vi "Main.vi"() -> ()   [LabVIEW 2024, in "Application.lvclass"]
uses:
  Application.lvclass
  <vilib>/event_ctls.llb/usereventprio.ctl
panel:
  in  "Button 20":bool
  in  "Button 19":bool
  in  "Button 18":bool
  in  "Button 17":bool
  in  "Button 16":bool
  in  "Button 15":bool
  in  "Button 14":bool
  in  "Button 13":bool
  in  "Button 12":bool
  in  "Button 11":bool
  in  "Button 10":bool
  in  "Button 9":bool
  in  "Button 8":bool
  in  "Button 7":bool
  in  "Button 6":bool
  in  "Button 5":bool
  in  "Button 4":bool
  in  "Button 3":bool
  in  "Button 2":bool
  in  "Button":bool
  out "User":string
  in  "Failure":bool
  in  "Next":bool
  in  "Previous":bool
  in  "Last":bool
  in  "First":bool
  out "date/time string":string
  in  "Tab Control":enum32{"Thumbnails", "Full Image", "Failures"}(tab)
  out "2D Picture 35":picture
  out "2D Picture 34":picture
  out "2D Picture 33":picture
  out "2D Picture 32":picture
  out "2D Picture 31":picture
  out "2D Picture 30":picture
  out "2D Picture 29":picture
  out "2D Picture 28":picture
  out "2D Picture 27":picture
  out "2D Picture 26":picture
  out "2D Picture 25":picture
  out "2D Picture 24":picture
  out "2D Picture 23":picture
  out "2D Picture 22":picture
  out "2D Picture 21":picture
  out "2D Picture 20":picture
  out "2D Picture 19":picture
  out "2D Picture 18":picture
  out "2D Picture 17":picture
  out "2D Picture 16":picture
  out "2D Picture 15":picture
  out "2D Picture 14":picture
  out "2D Picture 13":picture
  out "2D Picture 12":picture
  out "2D Picture 11":picture
  out "2D Picture 10":picture
  out "2D Picture 9":picture
  out "2D Picture 8":picture
  out "2D Picture":picture
  out "2D Picture 2":picture
  out "2D Picture 3":picture
  out "2D Picture 4":picture
  out "2D Picture 5":picture
  out "2D Picture 6":picture
  out "2D Picture 7":picture
  out "FullSize":picture
  out "error out":errorcluster
  # "IMAGE ANALYSIS PROTOTYPE"
  # "Hit any key to stop program"
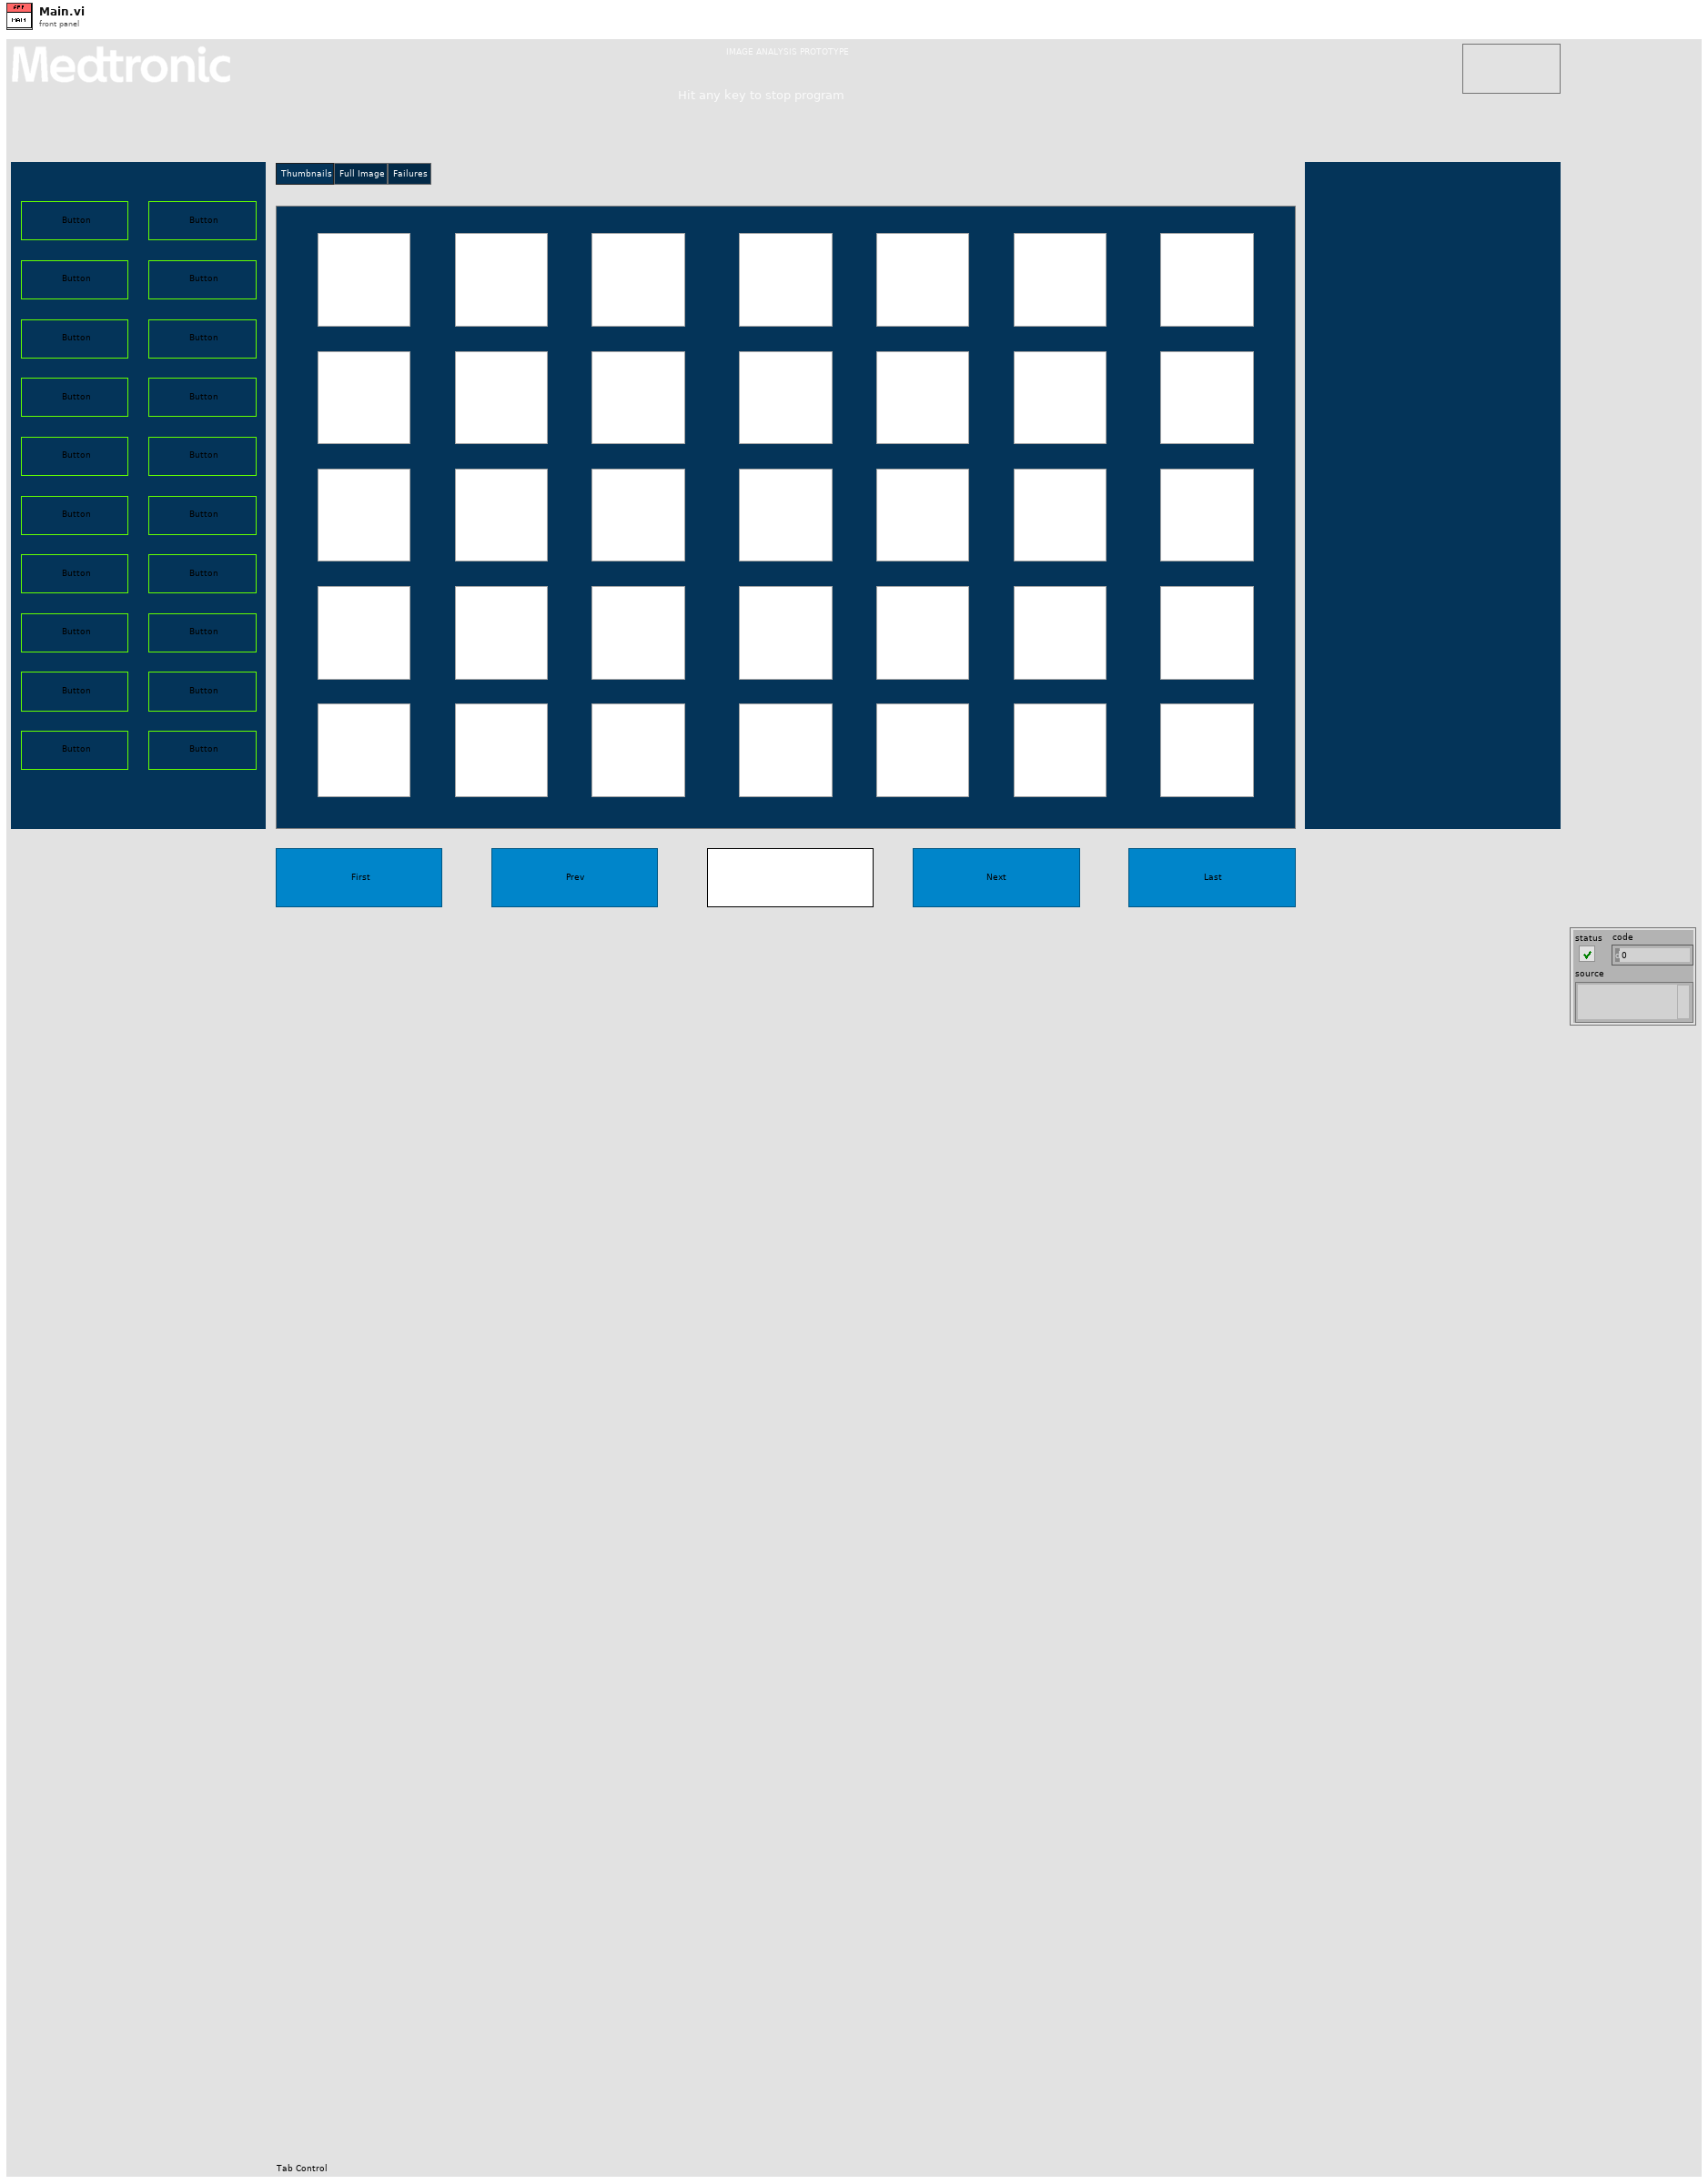
[diagram p1: front panel]
types:
  T1 = typedef "usereventprio.ctl" = enum32{"high priority", "normal priority"}
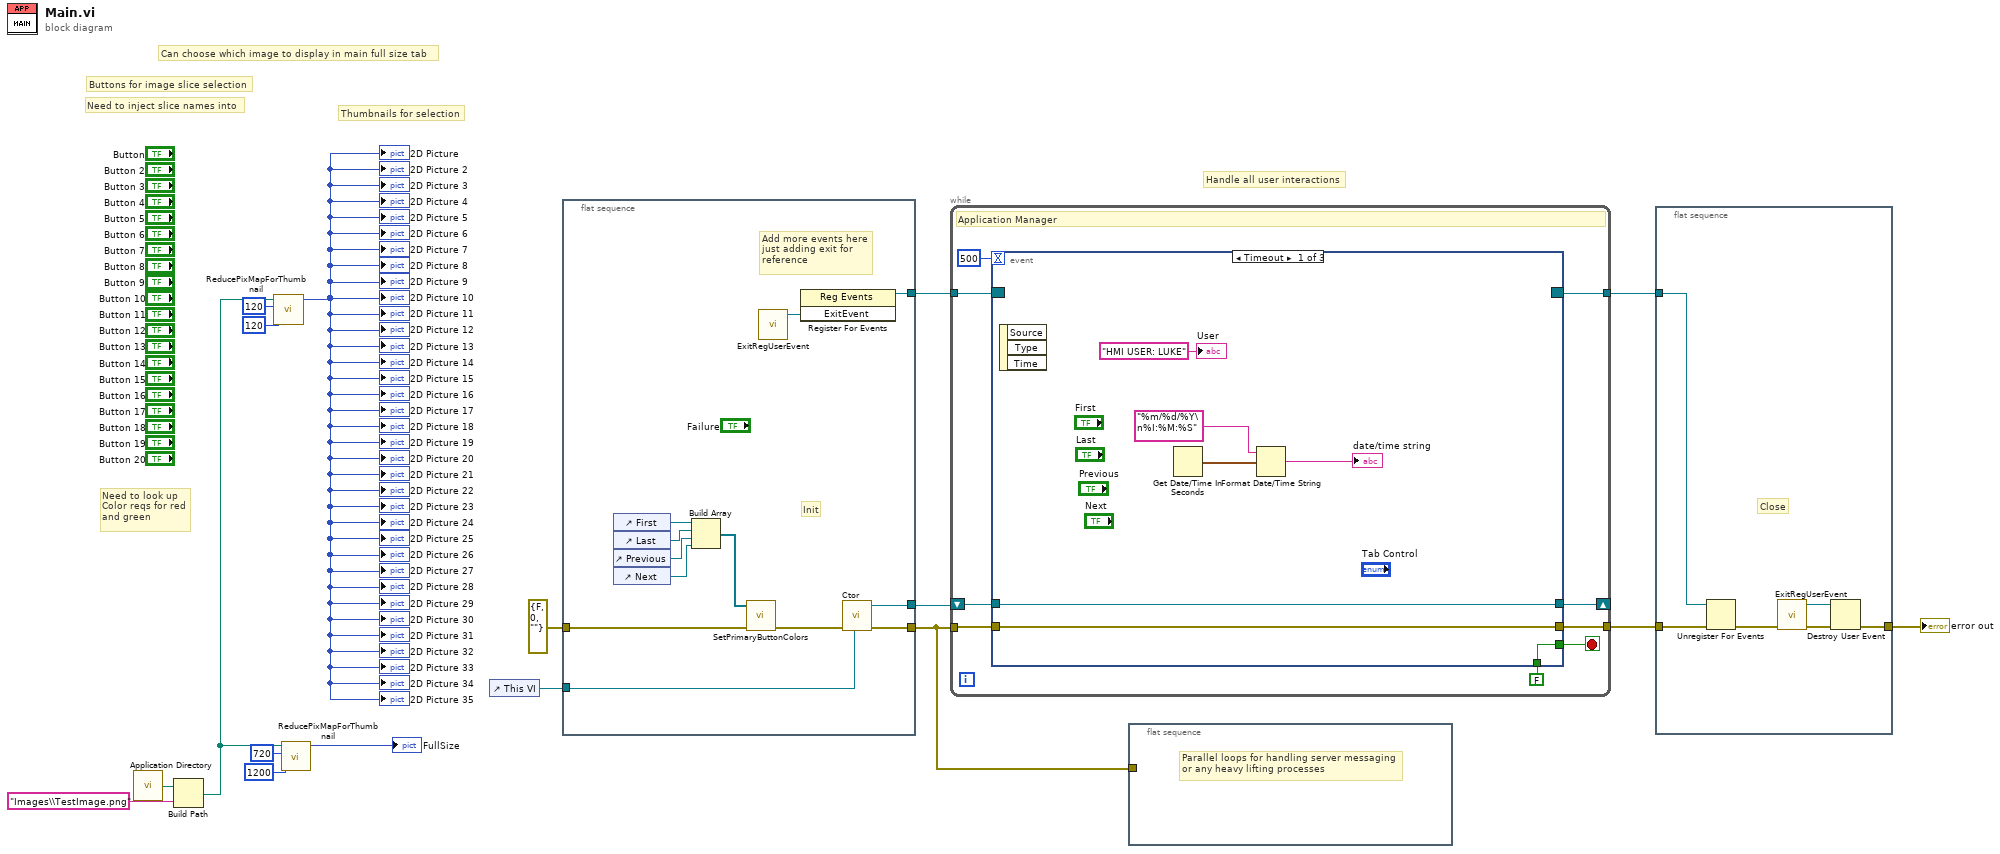
[diagram p0: block diagram]
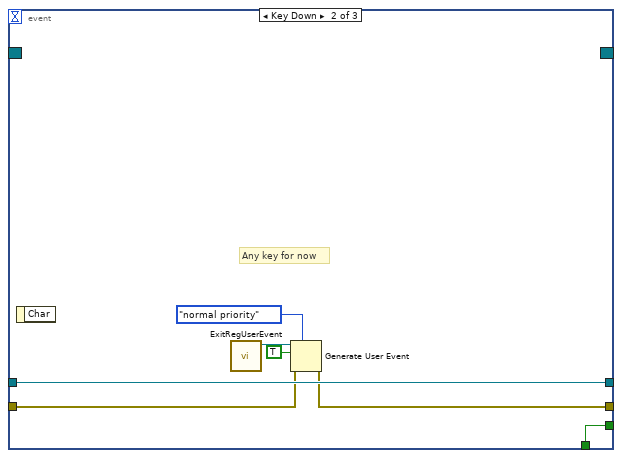
[diagram p2: hidden frame]
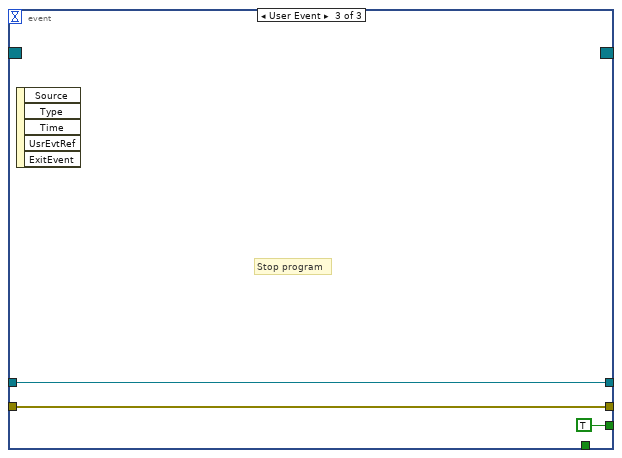
[diagram p3: hidden frame]
diagram:
  # "Handle all user interactions"
  # "Need to look up\nColor reqs for red\nand green"
  # "Need to inject slice names into"
  # "Can choose which image to display in main full size tab"
  # "Thumbnails for selection"
  # "Buttons for image slice selection"
  n1 = call <vilib>:"Application Directory.vi"() -> ("Application Directory"=w8:path)
  n2 = Build Path(base path=w8, name or relative path="Images\\TestImage.png") -> (appended path=w7:path)
  n3 = call "ReducePixMapForThumbnail.vi"("New Width"=120, "New Height"=120, "path to PNG file"=w7) -> ("new picture"=→"2D Picture" →"2D Picture 2" →"2D Picture 3" →"2D Picture 4" →"2D Picture 5" →"2D Picture 6" →"2D Picture 7" →"2D Picture 8" →"2D Picture 9" →"2D Picture 10" →"2D Picture 11" →"2D Picture 12" →"2D Picture 13" →"2D Picture 14" →"2D Picture 15" →"2D Picture 16" →"2D Picture 17" →"2D Picture 18" →"2D Picture 19" →"2D Picture 20" →"2D Picture 21" →"2D Picture 22" →"2D Picture 23" →"2D Picture 24" →"2D Picture 25" →"2D Picture 26" →"2D Picture 27" →"2D Picture 28" →"2D Picture 29" →"2D Picture 30" →"2D Picture 31" →"2D Picture 32" →"2D Picture 33" →"2D Picture 34" →"2D Picture 35":picture)  [unwired: 8 in]
  n4 = call "ReducePixMapForThumbnail.vi"("New Width"=1200, "New Height"=720, "path to PNG file"=w7) -> ("new picture"=→"FullSize":picture)  [unwired: 8 in]
  n5 = control-ref of="This VI"() -> (w16:refnum<vi>)
  n6 = flat-sequence {
    tunnel: errorcluster {"status"=FALSE, "code"=0, "source"=""} ("error in (no error)") -> [w18]
    tunnel: [w29] -> w1
    tunnel: w16 -> [w28]
    tunnel: [w27] -> w13
    tunnel: [w25] -> w11
    frame #0 {
      # "Add more events here\njust adding exit for\nreference"
      # "Init"
      n7 = control-ref of="First"() -> (w21:refnum<vi>)
      n8 = control-ref of="Last"() -> (w22:refnum<vi>)
      n9 = control-ref of="Previous"() -> (w23:refnum<vi>)
      n10 = control-ref of="Next"() -> (w24:refnum<vi>)
      n11 = Build Array(w21, w22, w23, w24) -> (w20:refnum<vi>[])
      n12 = call "SetPrimaryButtonColors.vi"("error in (no error)"=w18, "Booleans"=w20) -> ("error out"=w19:errorcluster)  [unwired: 9 in]
      n13 = call "ExitRegUserEvent.vi"() -> ("ExitEvent"=w26:refnum<user-event>)  [unwired: 11 in]
      n14 = register-events(w26) -> (reference out=w27:refnum<event-registration>)  [unwired: 2 in, 1 out]
      n15 = call "Ctor.vi"("This VI"=w28, "error in (no error)"=w19) -> ("error out"=w29:errorcluster, "Application out"=w25:refnum<class "Application.lvclass">)  [unwired: 8 in]
    }
  }
  n16 = while {
    tunnel: w1 -> [w37]
    tunnel: [w38] -> w15
    tunnel: w13 -> [w34]
    tunnel: [w33] -> w12
    shift-right: [w32] -> _
    shift-left: w11 -> [w31]
    stop <- w35 stop-if-true
    # "Application Manager"
    n17 = event shown="[0] Timeout" {
      selector: w34 -> [_ _ _]
      dyn-events: [_ _ _] -> w33
      timeout: 500 -> [_ _ _]
      tunnel: [w45 w50 w54] -> w38
      tunnel: w37 -> [w45 w51 w54]
      tunnel: FALSE -> [w44 w49 _]
      tunnel: [w44 w49 TRUE] -> w35
      tunnel: [w43 w52 w53] -> w32
      tunnel: w31 -> [w43 w52 w53]
      event Timeout {
        n18 = event-data() -> ()  [unwired: 1 in, 3 out]
        n19 = Get Date/Time In Seconds() -> (seconds since 1Jan1904=w42:timestamp)
        n20 = Format Date/Time String(time format string (%c)="%m/%d/%Y\n%I:%M:%S", seconds (now)=w42) -> (date/time string=→"date/time string":string)  [unwired: 1 in]
        "User" <- "HMI USER: LUKE" ("User")
      }
      event Key Down {
        # "Any key for now"
        n21 = event-data() -> ()  [unwired: 1 in, 1 out]
        n22 = call "ExitRegUserEvent.vi"() -> ("ExitEvent"=w48:refnum<user-event>)  [unwired: 11 in]
        n23 = Generate User Event(priority (normal)=usereventprio."normal priority", user event=w48, event data cluster=TRUE ("event data"), error in=w51) -> (error out=w50:errorcluster)  [unwired: 1 out]
      }
      event User Event {
        # "Stop program"
        n24 = event-data() -> ()  [unwired: 1 in, 5 out]
      }
    }
  }
  n25 = flat-sequence {
    tunnel: w1 -> [_]
    frame #0 {
      # "Parallel loops for handling server messaging\nor any heavy lifting processes"
    }
  }
  n26 = flat-sequence {
    tunnel: w15 -> [w60]
    tunnel: [w56] -> w14
    tunnel: w12 -> [w59]
    frame #0 {
      # "Close"
      n27 = Unregister For Events(event registration refnum=w59, error in=w60) -> (error out=w57:errorcluster)
      n28 = call "ExitRegUserEvent.vi"() -> ("ExitEvent"=w58:refnum<user-event>)  [unwired: 11 in]
      n29 = Destroy User Event(user event=w58, error in=w57) -> (error out=w56:errorcluster)
    }
  }
  "error out" <- w14
